vi "Get Device Parameter.vi"(8 "error in (no error)":errorcluster, 9 "Parameter Name":string, 10 "IED Name":string, 11 "SCADA in":refnum<class "SCADA.lvclass">) -> (0 "error out":errorcluster, 3 "SCADA out":refnum<class "SCADA.lvclass">)   [LabVIEW 2015, in "SCADA Core.lvlib" / "SCADA.lvclass"]
uses:
  SCADA.lvclass
  SCADA Abstract Messages/Get Device Parameter Status Msg/Get Device Parameter Status.ctl
  Utilities/Message Strings.llb/Data Type.ctl
  <vilib>/ActorFramework/Actor/Actor.lvclass/Actor.ctl
  SCADA.lvclass/SCADA.ctl
  <vilib>/ActorFramework/Actor/Actor.lvclass
  SCADA Abstract Messages/Get Device Parameter Status Msg/Get Device Parameter Status Msg.lvclass
  Utilities/Message Strings.llb/Message String Utilities.lvlib
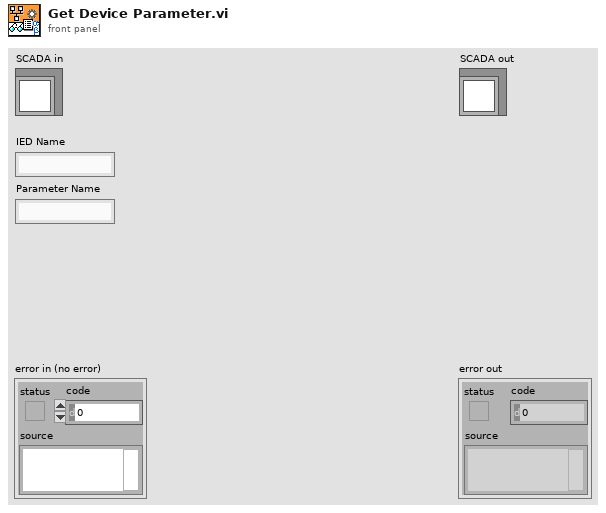
[diagram p1: front panel]
types:
  T1 = typedef "Message String Utilities.lvlib/Data Type.ctl" = enum16{"BOOL", "UINT8", "UINT32", "INT8", "INT32", "DBL", "STR"}
  T2 = enum16{"big-endian, network order", "native, host order", "little-endian"}
  T3 = typedef "SCADA Core.lvlib/Get Device Parameter Status Msg.lvclass/Get Device Parameter Status.ctl" = enum16{"Success", "Failure"}
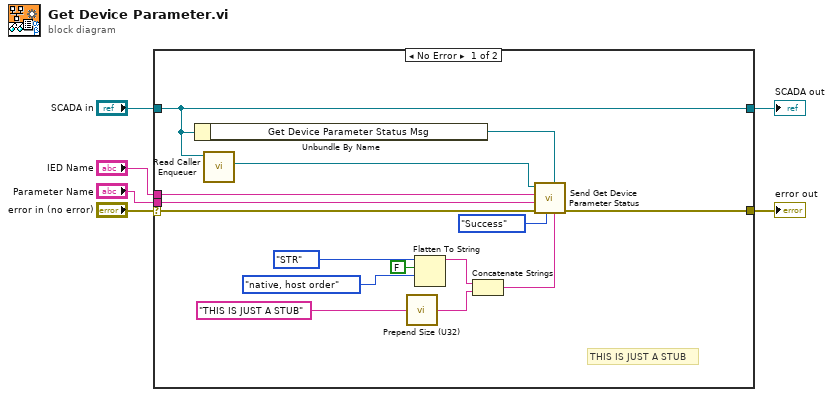
[diagram p0: block diagram]
diagram:
  n1 = case shown="No Error" "error in (no error)" {
    selector: "error in (no error)" -> [w17 w23]
    tunnel: [w15 w23] -> w5
    tunnel: [w21 w22] -> w3
    tunnel: "SCADA in" -> [w21 w22]
    tunnel: "IED Name" -> [w18 _]
    tunnel: "Parameter Name" -> [w16 _]
    frame No Error {
      # "THIS IS JUST A STUB"
      n2 = Unbundle By Name(w21) -> ("Get Device Parameter Status Msg"=w20:refnum<class "Get Device Parameter Status Msg.lvclass">)
      n3 = call <vilib>:"Read Caller Enqueuer.vi"("Actor"=w21) -> ("Caller Enqueuer"=w19:refnum<class "Message Enqueuer.lvclass">)  [unwired: 10 in]
      n4 = call "Prepend Size (U32).vi"("String in"="THIS IS JUST A STUB" ("error string")) -> ("String out"=w8:string)
      n5 = Flatten To String(anything=Data_Type."STR" ("Data Type"), prepend array or string size? (T)=FALSE, byte order (0:big-endian, network order)=T2."native, host order") -> (data string=w9:string)  [unwired: 1 in, 2 out]
      n6 = Concatenate Strings(w9, w8) -> (w7:string)
      n7 = call "Send Get Device Parameter Status.vi"("Parameter/Error"=w7, "Get Device Parameter Status Msg"=w20, "Status"=Get_Device_Parameter_Status."Success", "error in (no error)"=w17, "Parameter Name"=w16, "IED Name"=w18, "Message Enqueuer in"=w19) -> ("error out"=w15:errorcluster)  [unwired: 3 in, 1 out]
    }
    frame Error {
    }
  }
  "error out" <- w5
  "SCADA out" <- w3
